vi "From JSON Tree.vi"(8 "error in (no error)":errorcluster, 10 "JSON Tree In":variant, 11 "JSONable in":refnum<class "JSONable.lvclass">) -> (0 "error out":errorcluster, 3 "JSONable out":refnum<class "JSONable.lvclass">)   [LabVIEW 2015, in "JSONable.lvclass"]
uses:
  JSONable.lvclass
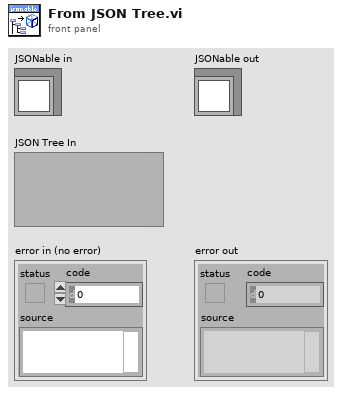
[diagram p1: front panel]
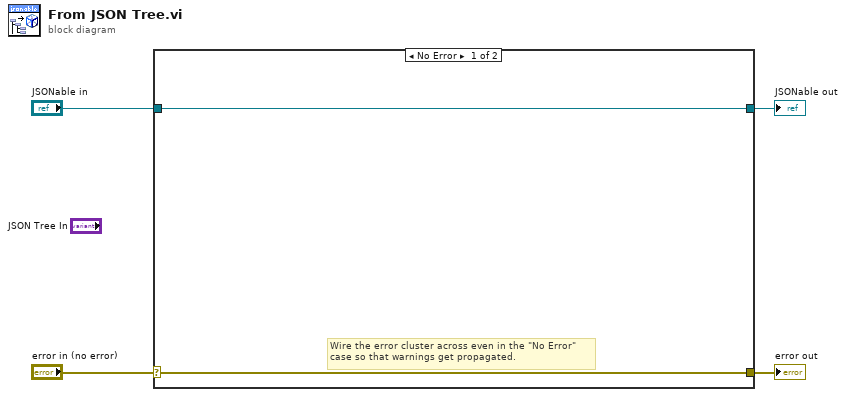
[diagram p0: block diagram]
diagram:
  n1 = case shown="No Error" "error in (no error)" {
    selector: "error in (no error)" -> [w6 w8]
    tunnel: [w6 w8] -> w3
    tunnel: [w5 w7] -> w1
    tunnel: "JSONable in" -> [w5 w7]
    frame No Error {
      # "Wire the error cluster across even in the \"No Error\"\ncase so that warnings get propagated."
    }
    frame Error {
    }
  }
  "error out" <- w3
  "JSONable out" <- w1
